vi "ParseKML.vi"(8 "error (in)":errorcluster, 11 ".kml File Path":path) -> (0 "error (out)":errorcluster, 3 "Waypoint Array":cluster{"Latitude":dbl, "Longitude":dbl}[](array[cluster]) {"Latitude" format="%#_15g"; "Longitude" format="%#_15g"})   [LabVIEW 2015]
doc: "Parses the incoming .kml file saved from Google Earth. Reads the latitude and longitude points in the document and saves them in a waypoint array to be used with the GPS."
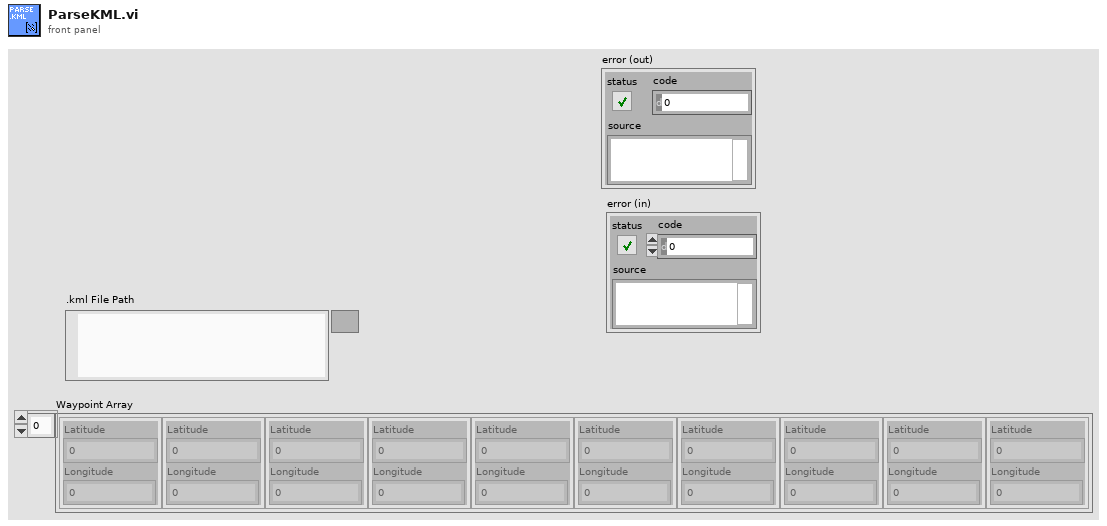
[diagram p1: front panel]
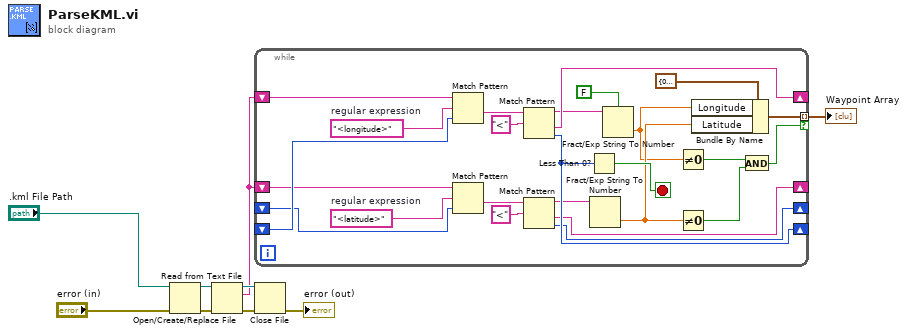
[diagram p0: block diagram]
diagram:
  n1 = Open/Create/Replace File(file path (use dialog)=".kml File Path", error in="error (in)") -> (refnum out=w8:refnum<file>, error out=w6:errorcluster)  [unwired: 2 in, 3 out]
  n2 = Read from Text File(file (use dialog)=w8, error in=w6) -> (refnum out=w7:refnum<file>, text=w2:string, error out=w5:errorcluster)  [unwired: 2 in, 1 out]
  n3 = while {
    shift-right: [w30] -> _
    shift-left: w2 -> [w31]
    shift-right: [w29] -> _
    shift-left: _ -> [w28]
    shift-right: [w22] -> _
    shift-left: w2 -> [w23]
    shift-right: [w21] -> _
    shift-left: _ -> [w20]
    tunnel: [w14] -> w3 mode=indexing if=w13
    stop <- w27 stop-if-true
    w24 = "<latitude>"  # regular expression
    w32 = "<longitude>"  # regular expression
    n4 = Match Pattern(string=w31, regular expression=w32, offset (0)=w28) -> (after substring=w34:string)  [unwired: 3 out]
    n5 = Match Pattern(string=w23, regular expression=w24, offset (0)=w20) -> (after substring=w25:string)  [unwired: 3 out]
    n6 = Match Pattern(string=w34, regular expression="<") -> (before substring=w12:string, after substring=w30:string, offset past match=w29:i32)  [unwired: 1 in, 1 out]
    n7 = Match Pattern(string=w25, regular expression="<") -> (before substring=w19:string, after substring=w22:string, offset past match=w21:i32)  [unwired: 1 in, 1 out]
    n8 = Less Than 0?(x=w29) -> (x < 0?=w27:bool)
    n9 = Fract/Exp String To Number(string=w19) -> (number=w17:dbl)  [unwired: 3 in, 1 out]
    n10 = Fract/Exp String To Number(use system decimal point (T)=FALSE, string=w12) -> (number=w11:dbl)  [unwired: 2 in, 1 out]
    n11 = Not Equal To 0?(x=w11) -> (x != 0?=w15:bool)
    n12 = Not Equal To 0?(x=w17) -> (x != 0?=w16:bool)
    n13 = Bundle By Name(cluster=cluster{"Latitude":dbl, "Longitude":dbl} {"Latitude"=0.0, "Longitude"=0.0} ("input cluster"), "Longitude"=w11, "Latitude"=w17) -> (w14:cluster{"Latitude":dbl, "Longitude":dbl})
    n14 = And(x=w15, y=w16) -> (x .and. y?=w13:bool)
  }
  "Waypoint Array" <- w3
  n15 = Close File(refnum=w7, error in=w5) -> (error out=→"error (out)":errorcluster)  [unwired: 1 out]
